vi "Data2UniqueID.vi"(7 "[UniqueID]s":string[](array[string]), 10 "ParameterSet":string, 11 "Step":string) -> (3 "UniqueID":string)   [LabVIEW 2013]
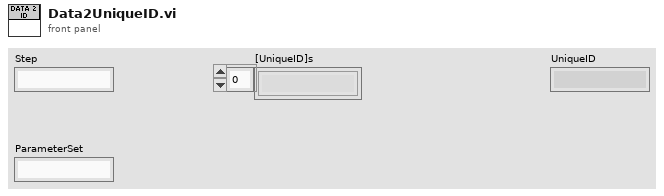
[diagram p1: front panel]
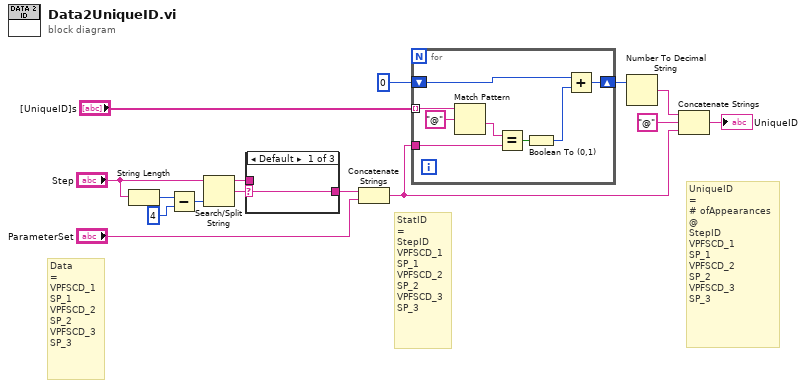
[diagram p0: block diagram]
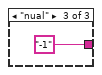
[diagram p3: hidden frame]
diagram:
  # "Data\n=\nVPFSCD_1\nSP_1\nVPFSCD_2\nSP_2\nVPFSCD_3\nSP_3"
  # "StatID\n=\nStepID\nVPFSCD_1\nSP_1\nVPFSCD_2\nSP_2\nVPFSCD_3\nSP_3"
  # "UniqueID\n=\n# ofAppearances\n@\nStepID\nVPFSCD_1\nSP_1\nVPFSCD_2\nSP_2\nVPFSCD_3\nSP_3"
  n1 = String Length(string="Step") -> (length=w13:i32)
  n2 = Subtract(x=w13, y=4) -> (x-y=w10:i32)
  n3 = Search/Split String(string="Step", offset (0)=w10) -> (substring before match=w9:string, match + rest of string=w11:string)  [unwired: 1 in, 1 out]
  n4 = case shown="Default" w11 {
    selector: w11 -> [w16 _ _]
    tunnel: [w16 w17 "-1"] -> w8
    tunnel: w9 -> [_ w17 _]
    frame Default {
    }
    frame " (M)" {
    }
    frame "nual" {
    }
  }
  n5 = Concatenate Strings(w8, "ParameterSet") -> (w3:string)
  n6 = for {
    tunnel: "[UniqueID]s" -> [w26] mode=indexing
    tunnel: w3 -> [w23]
    shift-right: [w21] -> w5
    shift-left: i16 0 -> [w22]
    n7 = Match Pattern(string=w26, regular expression="@") -> (after substring=w24:string)  [unwired: 1 in, 3 out]
    n8 = Equal?(x=w24, y=w23) -> (x = y?=w20:bool)
    n9 = Boolean To (0,1)(Boolean=w20) -> (0, 1=w19:i16)
    n10 = Add(x=w22, y=w19) -> (x+y=w21:i16)
  }
  n11 = Number To Decimal String(number=w5) -> (decimal integer string=w4:string)  [unwired: 1 in]
  n12 = Concatenate Strings(w4, "@" ("regular expression"), w3) -> (→"UniqueID":string)
